vi "Vision Research Phantom Series PhInt PhProcessImage.vi"(0 "pPixelSrc [in]":u16[](array[numeric]), 1 "IH [in]":T2, 2 "procID":T3 items=["IMG_PROC_REDUCE16TO8"=1], 3 "pProcParams":dbl, 5 "Error In (no error)":errorcluster) -> (14 "pPixelDest [out]":u8[](array[numeric]), 15 "IH [out]":T1, 19 "Error Out":errorcluster)   [LabVIEW 2013, in "VRI.lvlib"]
doc: "PhProcessImage\nvoid PhProcessImage(PBYTE pPixelSrc, PBYTE pPixelDest, PIH pIH, UINT procID, PVOID pProcParams);\n\nParameters\npPixelSrc [in]\n Input pixel data to be processed.\npPixelDest [out]\n Output buffer containing processed data.\npIH [in, out]\n Input: image header describing input data.\n Output: image header describing output data.\nprocID [in]\n Numerical value indicating the processing operation to be done. \npProcParams [in]\n Pointer to image processing parameters. \n\nReturn Value\nThe function returns ERR_Ok in case of success or an error code, otherwise. To get extended error information call PhGetErrorMessage.\n\nRemarks\nThe function processes the input cine as indicating by the numerical selector procID and according to pProcParams parameters.\npPixelSrc and pPixelDest may be identical, in which case, the operation is done in place.\n\nRequired Header\nPhInt.h"
uses:
  VRI.lvlib
  _Type Defs/PhInt PhProcessImage Selectors.ctl
  _Type Defs/PhInt IH.ctl
  Phantom DLLs/PhInt.Dll
panel:
  # "For instructions on the use of this VI, press Ctrl+H to display the help window and move the mouse over the icon, controls, and indicators"
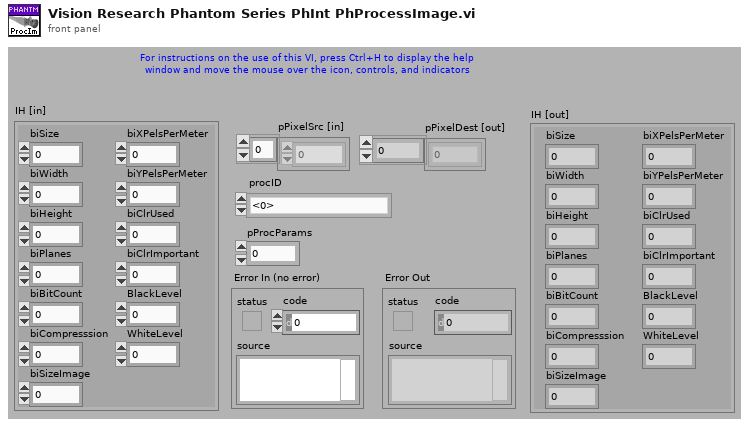
[diagram p1: front panel]
types:
  T1 = typedef "VRI.lvlib/PhInt IH.ctl" = cluster{"biSize":u32, "biWidth":i32, "biHeight":i32, "biPlanes":u16, "biBitCount":u16, "biCompresssion":u32, "biSizeImage":u32, "biXPelsPerMeter":i32, "biYPelsPerMeter":i32, "biClrUsed":u32, "biClrImportant":u32, "BlackLevel":i32, "WhiteLevel":i32}
  T2 = cluster{"biSize":u32, "biWidth":i32, "biHeight":i32, "biPlanes":u16, "biBitCount":u16, "biCompresssion":u32, "biSizeImage":u32, "biXPelsPerMeter":i32, "biYPelsPerMeter":i32, "biClrUsed":u32, "biClrImportant":u32, "BlackLevel":i32, "WhiteLevel":i32}
  T3 = typedef "VRI.lvlib/PhInt PhProcessImage Selectors.ctl" = u16
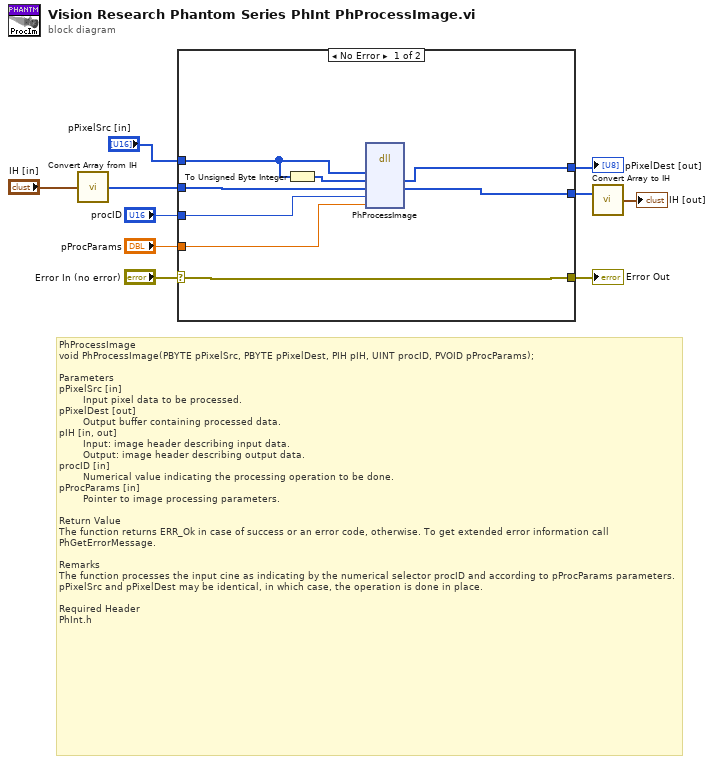
[diagram p0: block diagram]
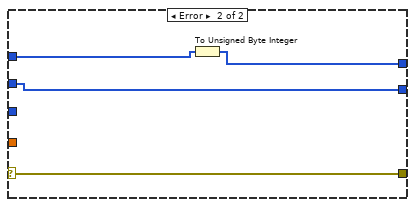
[diagram p2: hidden frame]
diagram:
  # "PhProcessImage\nvoid PhProcessImage(PBYTE pPixelSrc, PBYTE pPixelDest, PIH pIH, UINT procID, PVOID pProcParams);\n\nParameters\npPixelSrc [in]\n        Input pixel data to be processed.\npPixelDest [out]\n\t       Output buffer containing processed data.\npIH [in, out]\n\t       Input: image header describing input data.\n\t       Output: image header describing output data.\nprocID [in]\n        Numerical value indicating the processing operation to be done. \npProcParams [in]\n        Pointer to image processing parameters. \n\nReturn Value\nThe function returns ERR_Ok in case of success or an error code, otherwise. To get extended error information call PhGetErrorMessage.\n\nRemarks\nThe function processes the input cine as indicating by the numerical selector procID and according to pProcParams parameters.\npPixelSrc and pPixelDest may be identical, in which case, the operation is done in place.\n\nRequired Header\nPhInt.h"
  n1 = call "Convert Array from IH.vi"("IH"="IH [in]") -> ("Array"=w6:u8[])
  n2 = case shown="No Error" "Error In (no error)" {
    selector: "Error In (no error)" -> [w18 w22]
    tunnel: [w18 w22] -> w9
    tunnel: w6 -> [w17 w21]
    tunnel: "procID" -> [w16 _]
    tunnel: "pProcParams" -> [w15 _]
    tunnel: [w14 w21] -> w5
    tunnel: "pPixelSrc [in]" -> [w13 w20]
    tunnel: [w12 w19] -> w2
    frame No Error {
      n3 = To Unsigned Byte Integer(number=w13) -> (unsigned 8bit integer=w11:u8[])
      n4 = dll-call lib="C:/Projects/SDK/64-bit/Vision Research Phantom Series Labview Driver/Phantom DLLs/PhInt.dll" fn="PhProcessImage"("pPixelSrc"=w13, "pPixelDest"=w11, "pIH"=w17, "procID"=w16, "pProcParams"=w15) -> ("pPixelDest"=w12:u8[], "pIH"=w14:u8[])  [unwired: 4 in, 5 out]
    }
    frame Error {
      n5 = To Unsigned Byte Integer(number=w20) -> (unsigned 8bit integer=w19:u8[])
    }
  }
  "Error Out" <- w9
  "pPixelDest [out]" <- w2
  n6 = call "Convert Array to IH.vi"("Array"=w5) -> ("IH"=→"IH [out]":T1)
